vi "trans.vi"(1 "String":string) -> (0 "String 2":string)   [LabVIEW 2009]
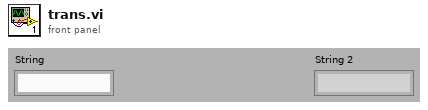
[diagram p1: front panel]
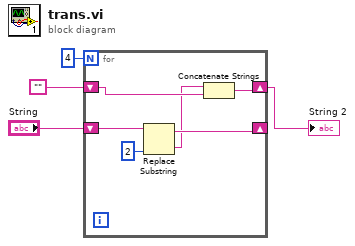
[diagram p0: block diagram]
diagram:
  n1 = for {
    N: 4 -> [_]
    shift-right: [w8] -> _
    shift-left: "String" -> [w10]
    shift-right: [w5] -> w1
    shift-left: "" -> [w7]
    n2 = Replace Substring(2:2 ("length (len. of substring)"), 5:w10) -> (0:w6:string, 1:w8:string)  [unwired: 2 in]
    n3 = Concatenate Strings(w6, w7) -> (w5:string)
  }
  "String 2" <- w1
